vi "Read Time.vi"(8 "error in (no error)":errorcluster, 11 "9213 in":refnum<class "9213.lvclass">) -> (0 "error out":errorcluster, 2 "Conversion Time":T1=1 items=["High Speed", "High Resolution"], 3 "9213 out":refnum<class "9213.lvclass">)   [LabVIEW 2017, in "Modules.lvlib" / "9213.lvclass"]
uses:
  9213.lvclass
  Conversion Time.ctl
  9213.lvclass/9213.ctl
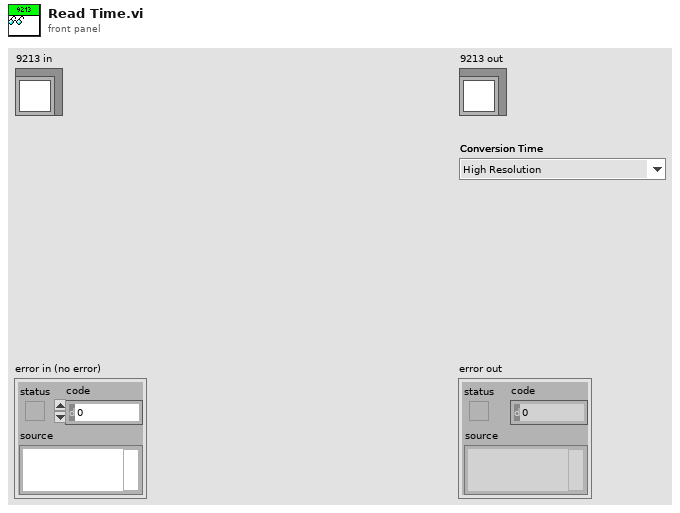
[diagram p1: front panel]
types:
  T1 = typedef "Modules.lvlib/9213.lvclass/Conversion Time.ctl" = u16
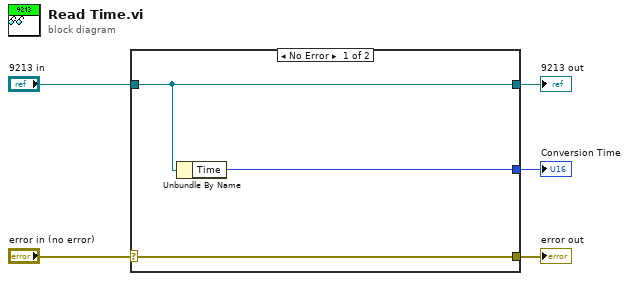
[diagram p0: block diagram]
diagram:
  n1 = case shown="No Error" "error in (no error)" {
    selector: "error in (no error)" -> [w8 w9]
    tunnel: [w8 w9] -> w4
    tunnel: [w7 w10] -> w2
    tunnel: "9213 in" -> [w7 w10]
    tunnel: [w6 _] -> w1
    frame No Error {
      n2 = Unbundle By Name(w7) -> ("Time"=w6:T1)
    }
    frame Error {
    }
  }
  "error out" <- w4
  "9213 out" <- w2
  "Conversion Time" <- w1
